vi "AKIP_error_check.vi"(8 "error in (no error)":errorcluster, 11 "VISA Refnum in":refnum<visa-resource-name>="AKIP") -> (0 "error out":errorcluster, 3 "VISA Refnum out":refnum<visa-resource-name>)   [LabVIEW 2017]
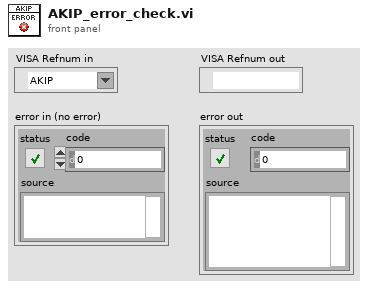
[diagram p1: front panel]
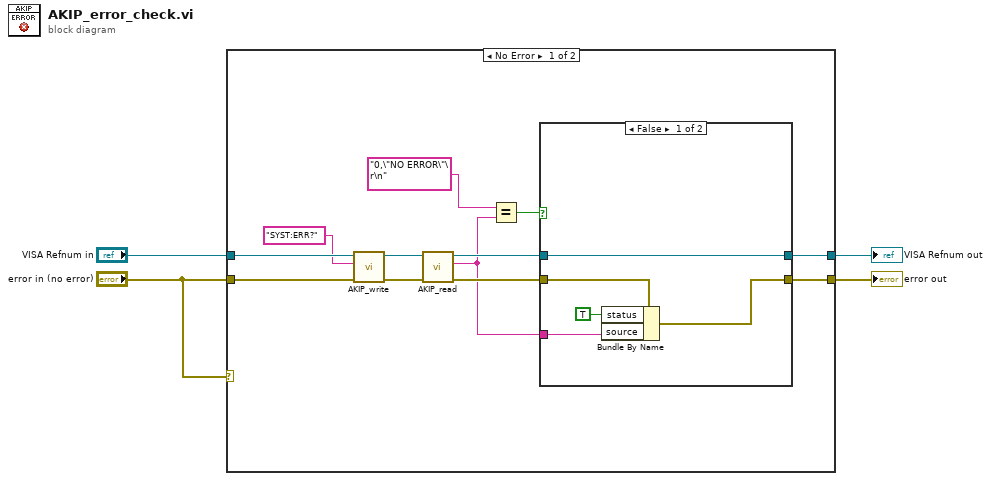
[diagram p0: block diagram]
diagram:
  n1 = case shown="No Error" "error in (no error)" {
    tunnel: [w15 w24] -> w4
    tunnel: [w14 w25] -> w3
    tunnel: "VISA Refnum in" -> [w9 w25]
    tunnel: "error in (no error)" -> [w10 w24]
    frame No Error {
      n2 = call "AKIP_write.vi"("error in (no error)"=w10, "write buffer"="SYST:ERR?", "VISA Refnum in"=w9) -> ("error out"=w11:errorcluster, "VISA Refnum out"=w12:refnum<visa-resource-name>)  [unwired: 7 in]
      n3 = call "AKIP_read.vi"("error in (no error)"=w11, "VISA Refnum in"=w12) -> ("error out"=w8:errorcluster, "read buffer"=w5:string, "VISA Refnum out"=w7:refnum<visa-resource-name>)  [unwired: 7 in]
      n4 = Equal?(x="0,\"NO ERROR\"\r\n" ("read buffer 2"), y=w5) -> (x = y?=w16:bool)
      n5 = case shown="False" w16 {
        tunnel: w8 -> [w21 w22]
        tunnel: w7 -> [w18 w23]
        tunnel: [w18 w23] -> w14
        tunnel: [w20 w22] -> w15
        tunnel: w5 -> [w17 _]
        frame False {
          n6 = Bundle By Name(cluster=w21, "status"=TRUE, "source"=w17) -> (w20:errorcluster)
        }
        frame True {
        }
      }
    }
    frame Error {
    }
  }
  "VISA Refnum out" <- w3
  "error out" <- w4
